vi "convert_string_to_booleanArray.vi"(2 "Max Elements Count (All)":i32=-1, 4 "String in":string) -> (0 "boolean array size":i32 caption="string array size", 1 "boolean array out":bool[](array[boolean]))   [LabVIEW 2014, in "rszvl_rsidr_core.lvlib"]
uses:
  rszvl_rsidr_core.lvlib
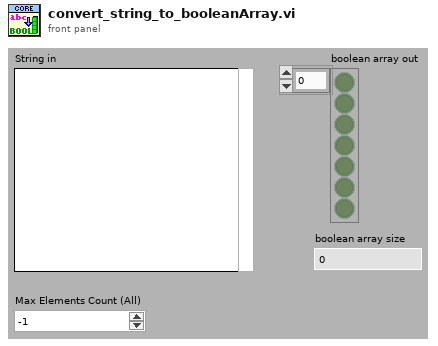
[diagram p1: front panel]
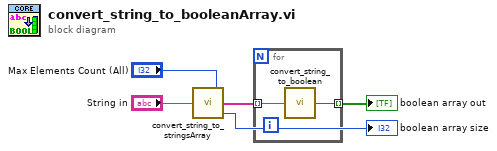
[diagram p0: block diagram]
diagram:
  n1 = call "convert_string_to_stringsArray.vi"("Max Elements Count (All)"="Max Elements Count (All)", "String in"="String in") -> ("string array size out"=→"boolean array size":i32, "string array out"=w3:string[])  [unwired: 2 in]
  n2 = for {
    tunnel: w3 -> [w7] mode=indexing
    tunnel: [w6] -> w5 mode=indexing
    n3 = call "convert_string_to_boolean.vi"("String in"=w7) -> ("boolean value out"=w6:bool)  [unwired: 4 in]
  }
  "boolean array out" <- w5
